vi "Close Nested.vi"(8 "error in (no error)":errorcluster, 10 "Nested":T1, 11 "Open Close Logic in":refnum<class "Open Close Logic.lvclass">) -> (0 "error out":errorcluster, 3 "Open Close Logic out":refnum<class "Open Close Logic.lvclass">)   [LabVIEW 2020, in "Form Server Interfaces.lvlib" / "Open Close Logic.lvclass"]
uses:
  Open Close Logic.lvclass
  Form ID.ctl
  Form Server Interfaces.lvlib
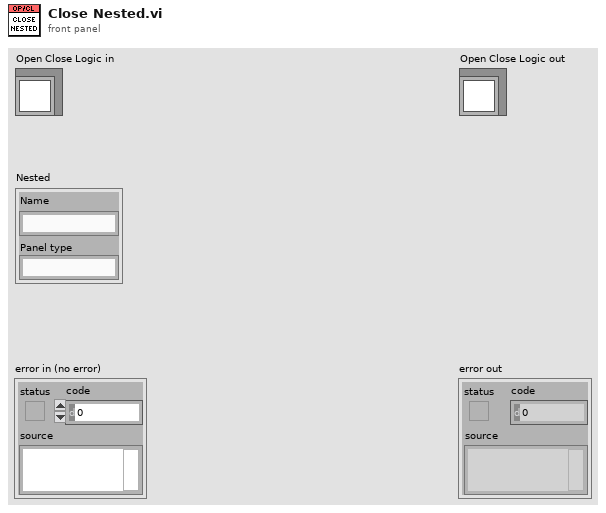
[diagram p1: front panel]
types:
  T1 = typedef "Form Server Interfaces.lvlib/Form ID.ctl" = cluster{"Name":string, "Panel type":string}
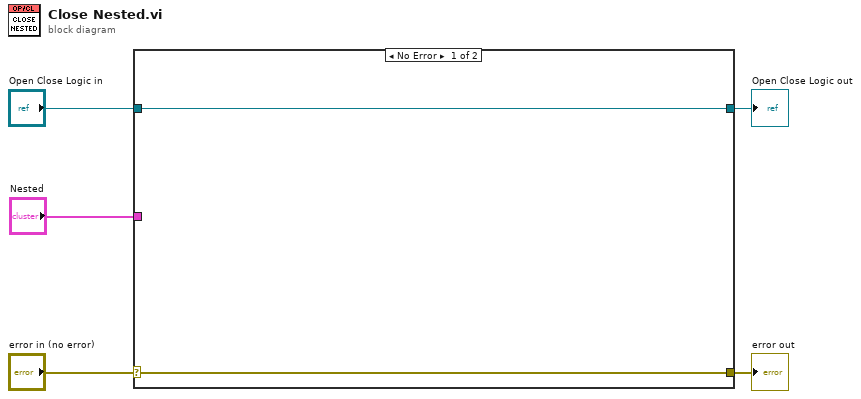
[diagram p0: block diagram]
diagram:
  n1 = case shown="No Error" "error in (no error)" {
    selector: "error in (no error)" -> [w7 w9]
    tunnel: [w7 w9] -> w4
    tunnel: [w6 w8] -> w2
    tunnel: "Open Close Logic in" -> [w6 w8]
    tunnel: "Nested" -> [_ _]
    frame No Error {
    }
    frame Error {
    }
  }
  "error out" <- w4
  "Open Close Logic out" <- w2
